vi "find_midpoint_retroreflective.vi"(1 "Cluster":T1, 2 "run_time":fxp<+,40,40>) -> (0 "timeOfMidpoint":fxp<+,41,40>)   [LabVIEW 2018]
uses:
  comp-src/validated_bool.ctl
  <vilib>/rvi/FXPMathLib/FxpAdd/XNode/nifxpmath_Add.xnode
  <vilib>/rvi/FXPMathLib/FxpMul/XNode/nifxpmath_Multiplier.xnode
  <vilib>/rvi/FXPMathLib/sim/FxpSim.dll
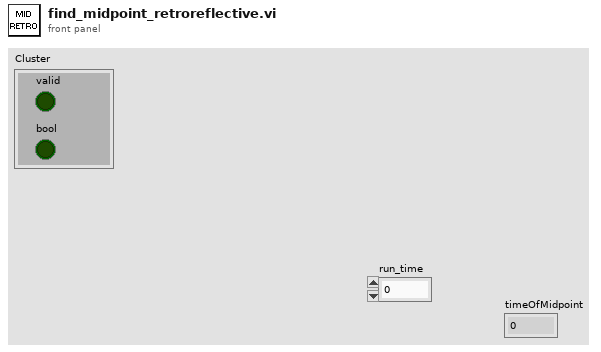
[diagram p1: front panel]
types:
  T1 = typedef "validated_bool.ctl" = cluster{"valid":bool, "bool":bool}
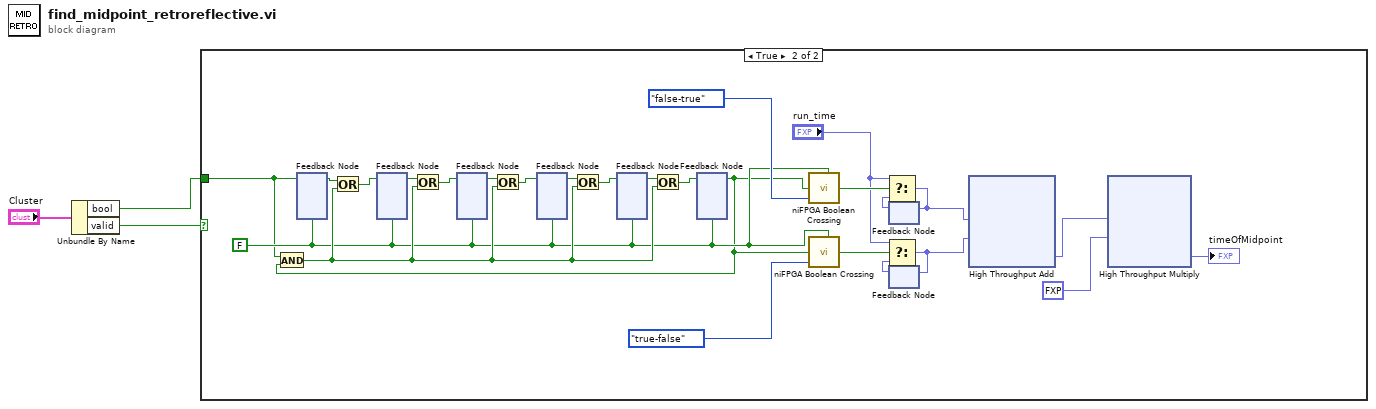
[diagram p0: block diagram]
diagram:
  n1 = Unbundle By Name("Cluster") -> ("bool"=w1:bool, "valid"=w2:bool)
  n2 = case shown="True" w2 {
    tunnel: w1 -> [_ w4]
    frame False {
    }
    frame True {
      w17 = FALSE
      n3 = feedback #1(w17) -> (w29:bool)
      n4 = feedback-in #1(w4) -> ()
      n5 = feedback #2(w17) -> (w28:bool)
      n6 = feedback #3(w17) -> (w27:bool)
      n7 = feedback #4(w17) -> (w26:bool)
      n8 = feedback #5(w17) -> (w22:bool)
      n9 = feedback #6(w17) -> (w16:bool)
      n10 = And(x=w4, y=w16) -> (x .and. y?=w19:bool)
      n11 = Or(x=w29, y=w19) -> (x .or. y?=w23:bool)
      n12 = feedback-in #2(w23) -> ()
      n13 = Or(x=w28, y=w19) -> (x .or. y?=w24:bool)
      n14 = feedback-in #3(w24) -> ()
      n15 = Or(x=w27, y=w19) -> (x .or. y?=w25:bool)
      n16 = feedback-in #4(w25) -> ()
      n17 = Or(x=w26, y=w19) -> (x .or. y?=w21:bool)
      n18 = feedback-in #5(w21) -> ()
      n19 = Or(x=w22, y=w19) -> (x .or. y?=w20:bool)
      n20 = feedback-in #6(w20) -> ()
      n21 = call <vilib>:"niFPGA Boolean Crossing.vi"("input"=w16, "direction"=enum8{"either", "false-true", "true-false"}."false-true", "initialize"=w17) -> ("crossing"=w15:bool)  [unwired: 6 in]
      n22 = call <vilib>:"niFPGA Boolean Crossing.vi"("input"=w16, "direction"=enum8{"either", "false-true", "true-false"}."true-false", "initialize"=w17) -> ("crossing"=w14:bool)  [unwired: 6 in]
      n23 = feedback #7() -> (w12:fxp<+,40,40>)  [unwired: 1 in]
      n24 = Select(t="run_time", s=w15, f=w12) -> (s? t:f=w9:fxp<+,40,40>)
      n25 = feedback-in #7(w9) -> ()
      n26 = feedback #8() -> (w13:fxp<+,40,40>)  [unwired: 1 in]
      n27 = Select(t="run_time", s=w14, f=w13) -> (s? t:f=w8:fxp<+,40,40>)
      n28 = feedback-in #8(w8) -> ()
      n29 = xnode "High Throughput Add"("x"=w9, "y"=w8) -> ("x+y"=w7:fxp<+,41,41>)
      n30 = xnode "High Throughput Multiply"("x"=w7, "y"=fxp<+,1,0> 0.5) -> ("x*y"=→"timeOfMidpoint":fxp<+,41,40>)
    }
  }
